vi "LS372_setup.vi"() -> (0 "error out":errorcluster caption="Fehler (Ausgang)")   [LabVIEW 2019]
uses:
  Instrument_Setup.vi
  Global/Global Variables/Data_Display_global.vi
  Equipment/Lake Shore 372/Lake Shore 372.lvlib
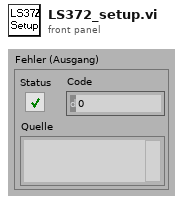
[diagram p1: front panel]
types:
  T1 = typedef "LS372-Cluster.ctl" = cluster{"Activate Tsweep":bool, "Setpoint - Manual":dbl, "Rate (K/min)":dbl, "Update Lakeshores":bool, "Still Heater":bool, "Still Power (mW)":dbl, "Manual Heater":bool, "Manual Heater  (mW) ":dbl, "Heater Range":dbl, "P (Gain)":dbl, "I (Reset)":dbl, "D (Rate)":dbl, "Heater Power (mW)":dbl, "MC Thermometer":u16, "MC Temperature":dbl, "LS372-T1":dbl, "LS372 -T2":dbl, "LS372-R1 ":dbl, "LS372-R2":dbl, "LS372-T3":dbl, "LS372-T4":dbl, "LS372-R3 ":dbl, "LS372-R4 \n\n\n\n":dbl, "LS372-T5":dbl, "LS372-T6":dbl, "LS372-R5":dbl, "LS372-R6 ":dbl, "Still Power ist":dbl, "Set Temperatur Sweep main":bool, "Setpoint ist":dbl, "Disable Heater":bool}
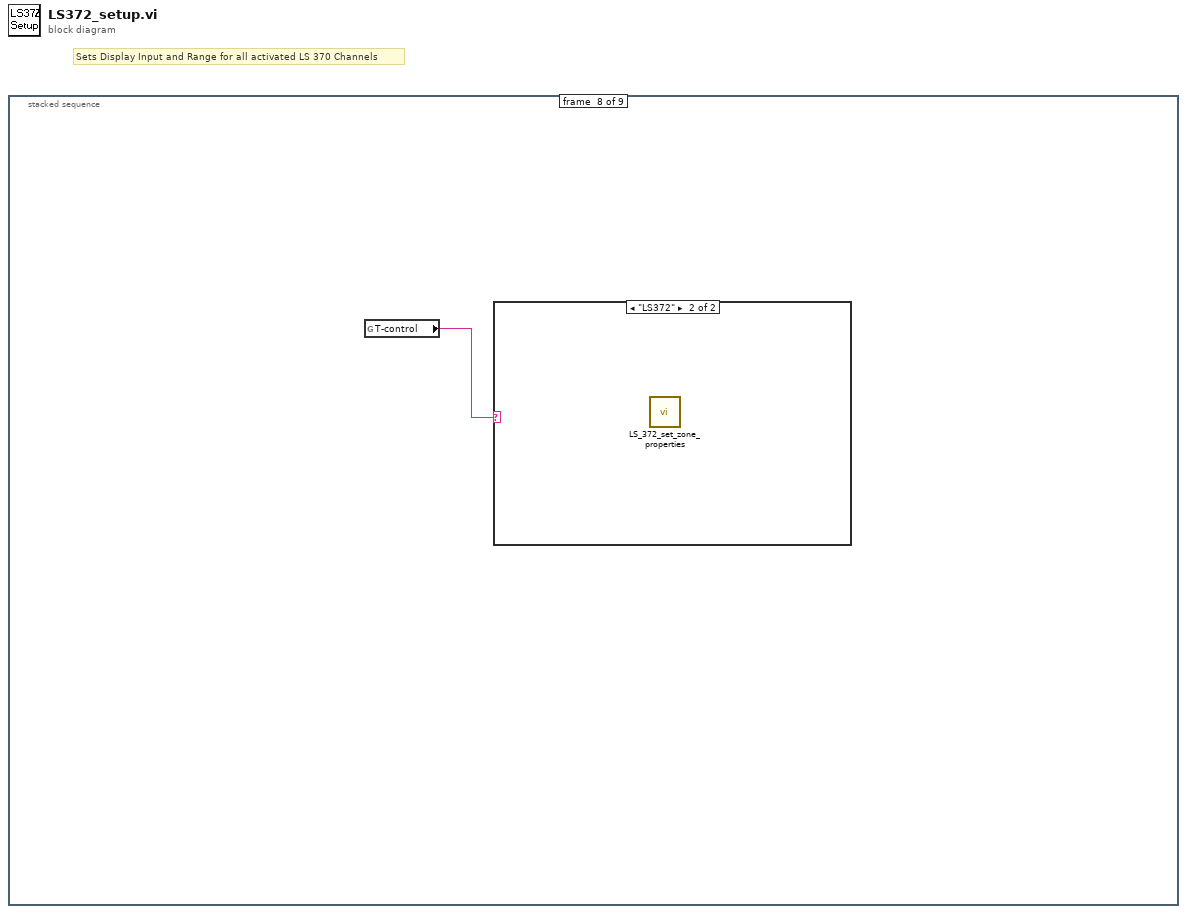
[diagram p0: block diagram]
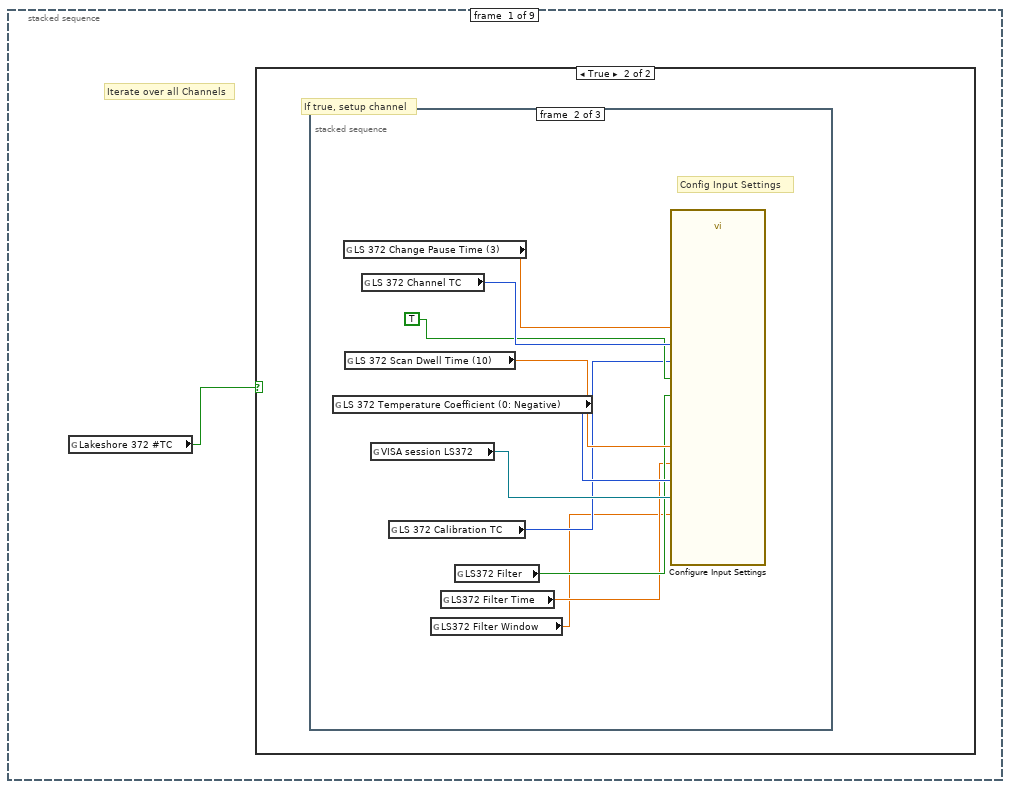
[diagram p2: hidden frame]
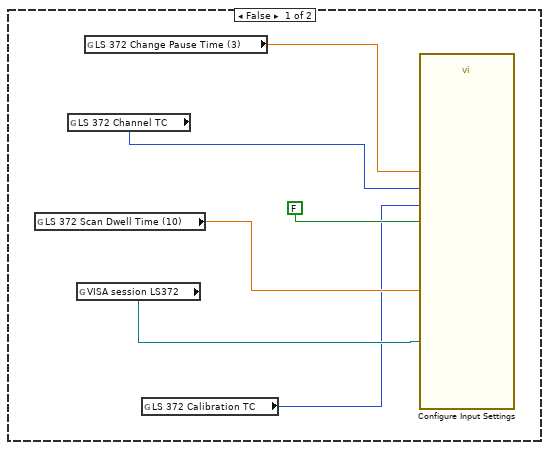
[diagram p3: hidden frame]
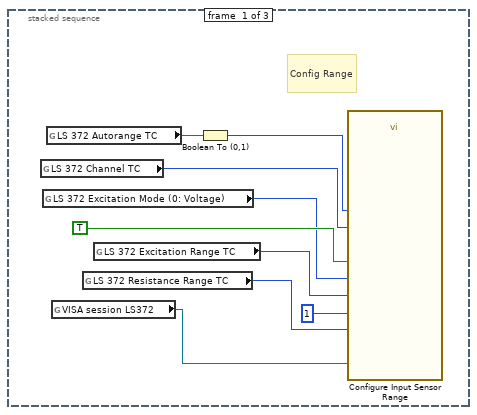
[diagram p4: hidden frame]
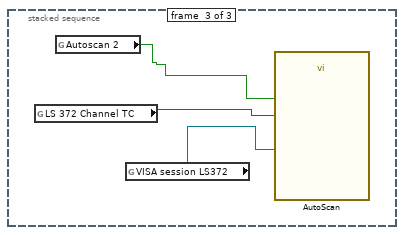
[diagram p5: hidden frame]
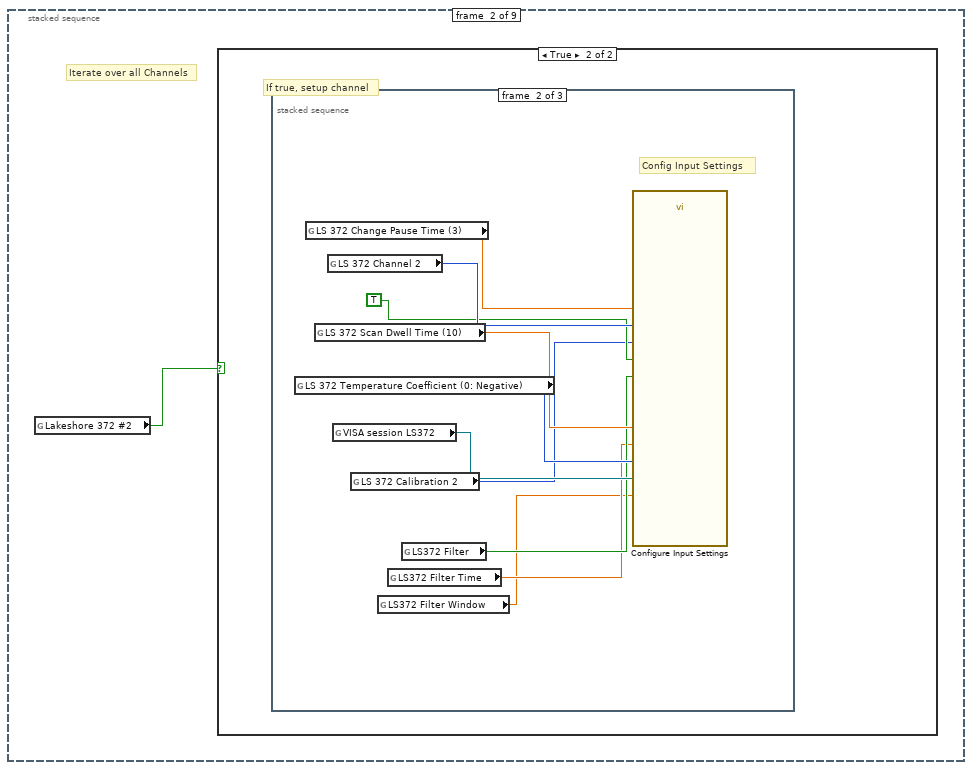
[diagram p6: hidden frame]
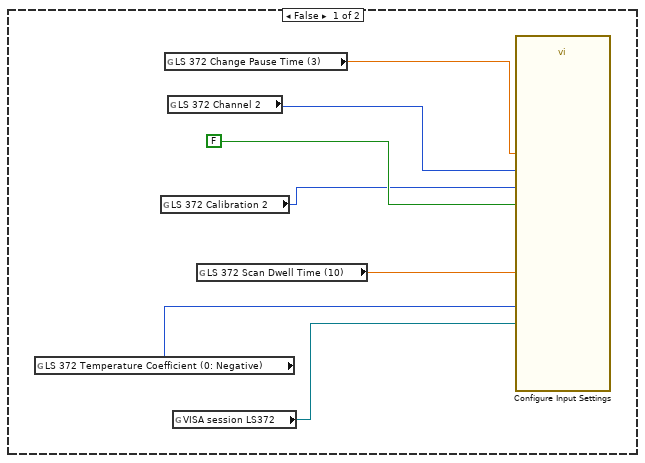
[diagram p7: hidden frame]
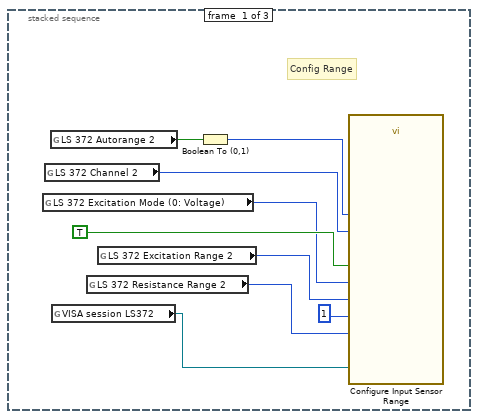
[diagram p8: hidden frame]
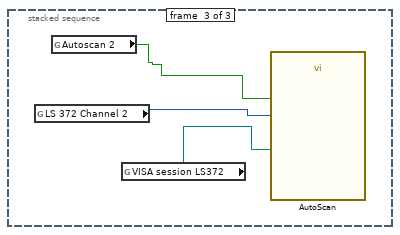
[diagram p9: hidden frame]
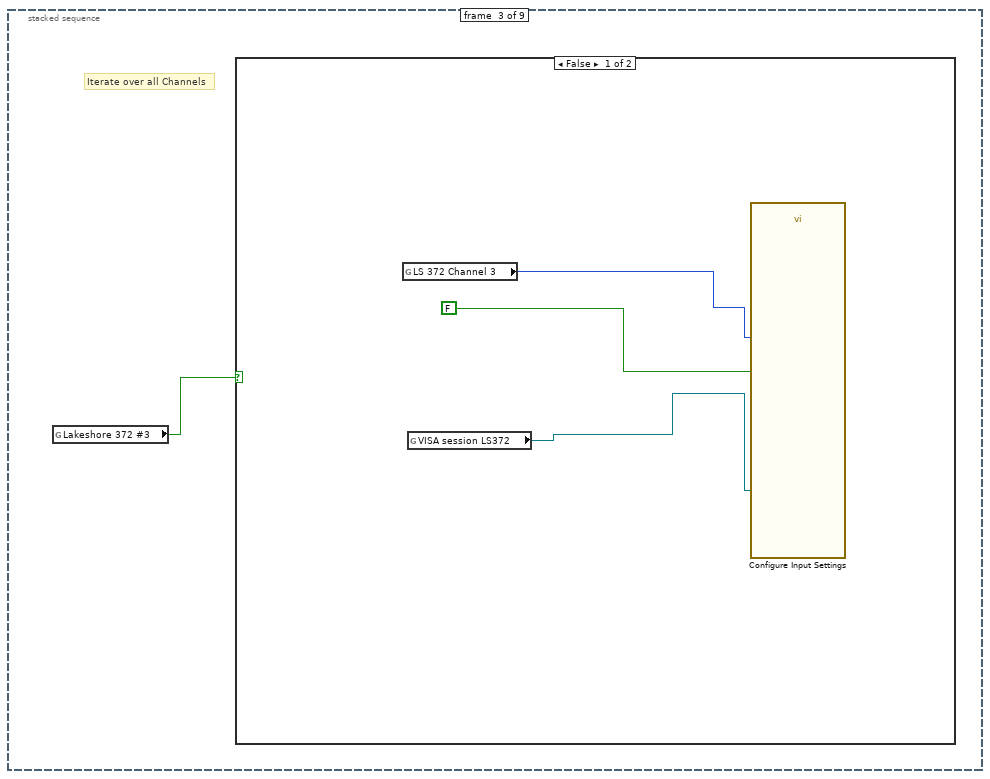
[diagram p10: hidden frame]
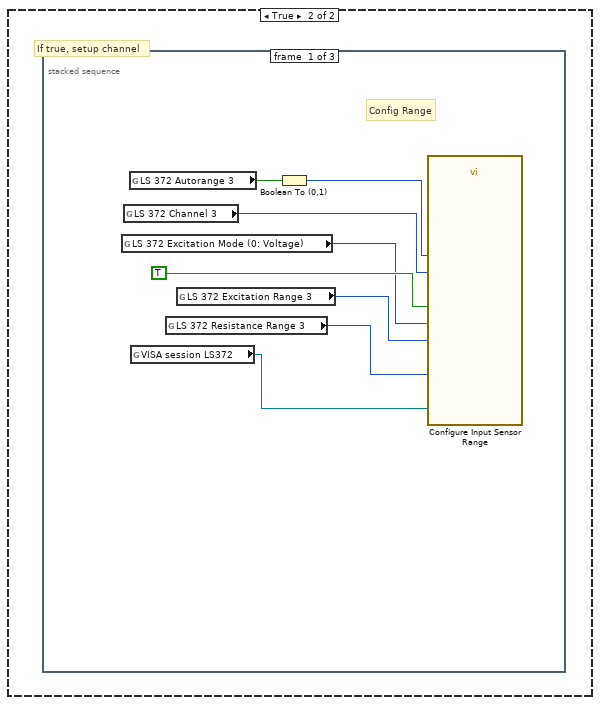
[diagram p11: hidden frame]
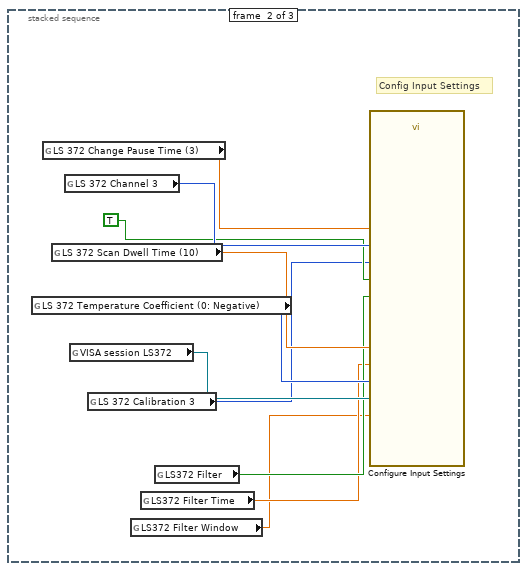
[diagram p12: hidden frame]
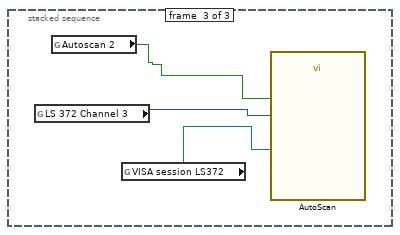
[diagram p13: hidden frame]
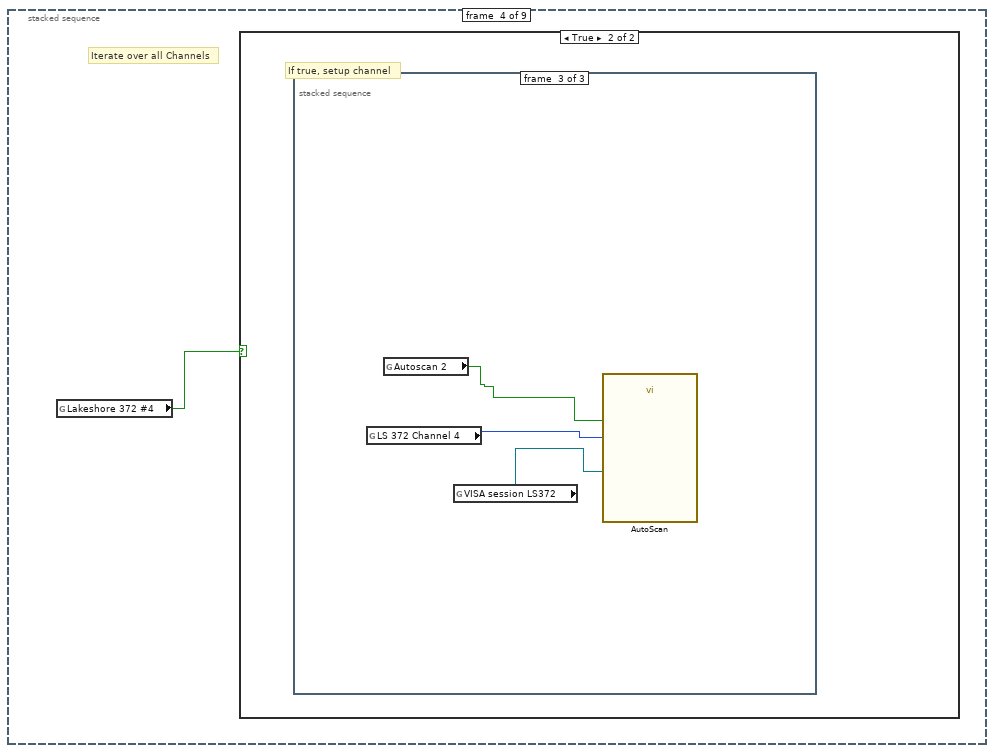
[diagram p14: hidden frame]
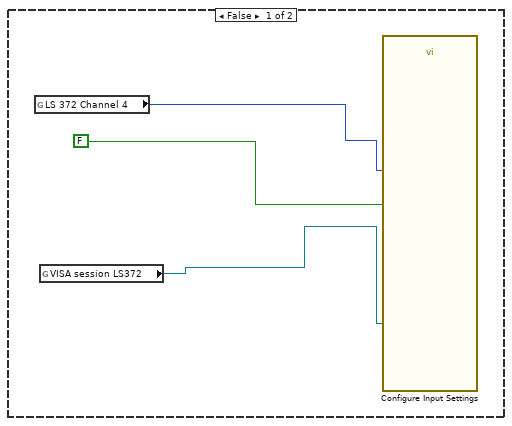
[diagram p15: hidden frame]
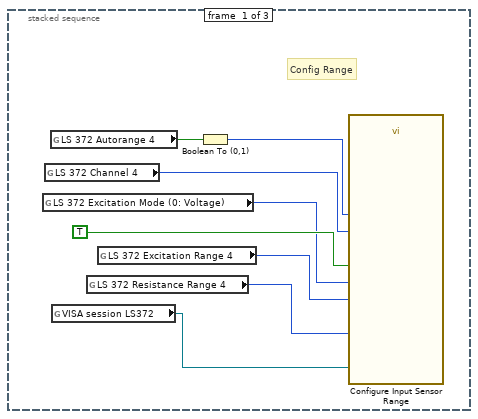
[diagram p16: hidden frame]
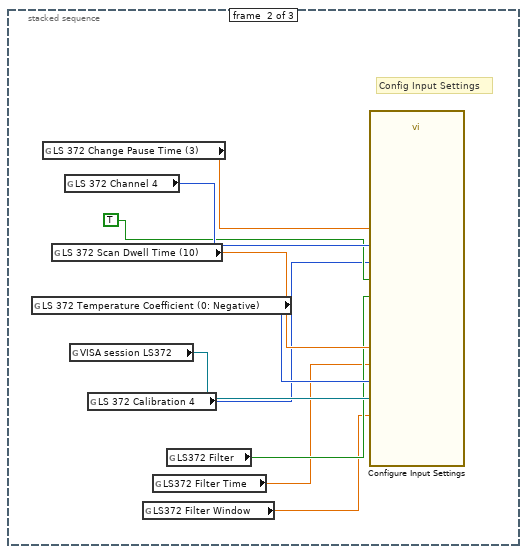
[diagram p17: hidden frame]
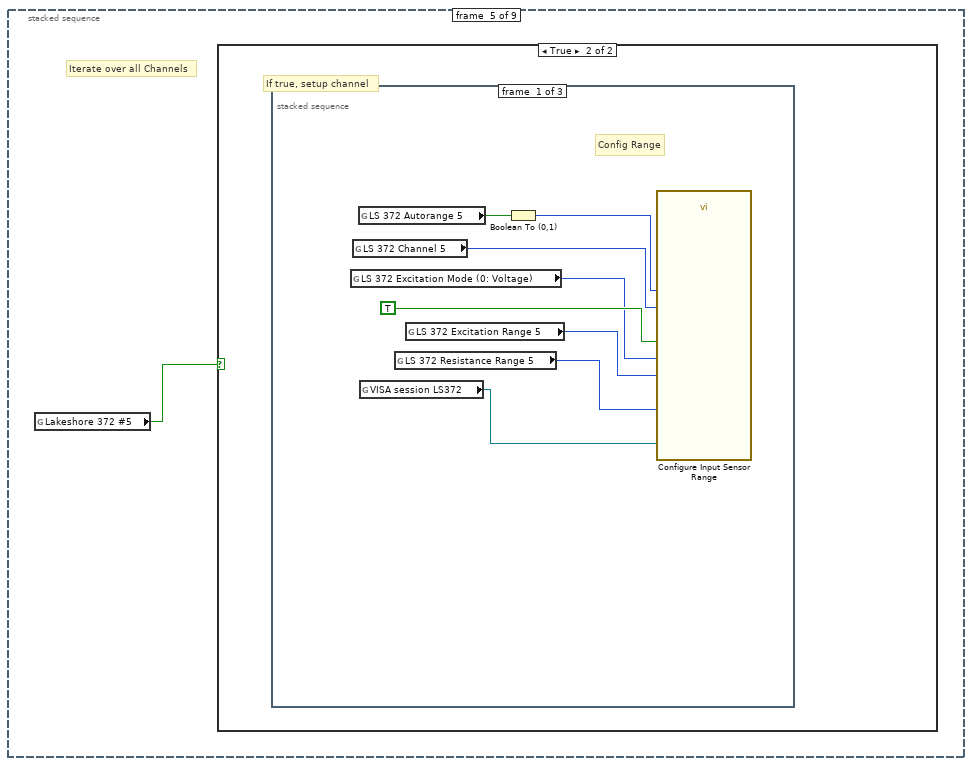
[diagram p18: hidden frame]
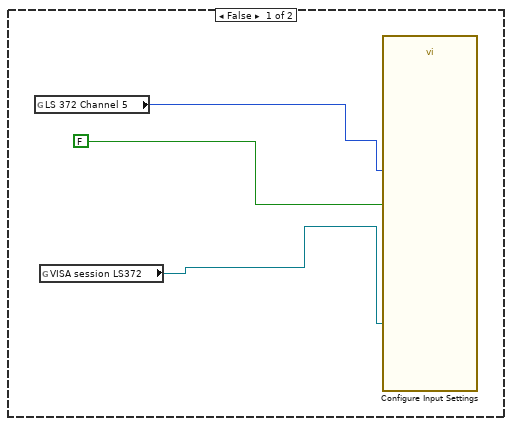
[diagram p19: hidden frame]
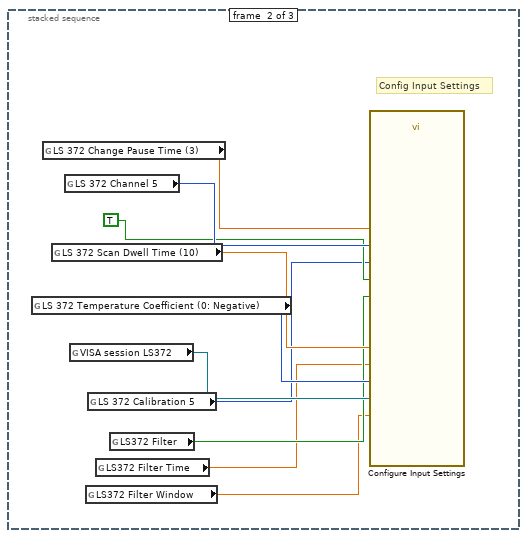
[diagram p20: hidden frame]
diagram:
  # "Sets Display Input and Range for all activated LS 370 Channels"
  n1 = stacked-sequence {
    frame #0 {
      # "Iterate over all Channels"
      n2 = global read "Instrument_Setup.vi" "Lakeshore 372 #TC"() -> (w1:bool)
      n3 = case shown="True" w1 {
        frame False {
          n4 = global read "Instrument_Setup.vi" "LS 372 Scan Dwell Time (10)"() -> (w3:dbl)
          n5 = global read "Instrument_Setup.vi" "LS 372 Channel TC"() -> (w7:u16)
          n6 = global read "Instrument_Setup.vi" "VISA session LS372"() -> (w5:refnum<visa-resource-name>)
          n7 = global read "Instrument_Setup.vi" "LS 372 Change Pause Time (3)"() -> (w4:dbl)
          n8 = global read "Instrument_Setup.vi" "LS 372 Calibration TC"() -> (w2:i32)
          n9 = call "Configure Input Settings.vi"("VISA resource name"=w5, "Channel (1)"=w7, "Scan Dwell Time (10)"=w3, "Change Pause Time (3)"=w4, "Curve Number (0)"=w2, "Enable Channel (T: Enable)"=FALSE) -> ()  [unwired: 12 in, 2 out]
        }
        frame True {
          # "If true, setup channel"
          n10 = stacked-sequence {
            frame #0 {
              # "Config Range"
              n11 = global read "Instrument_Setup.vi" "LS 372 Channel TC"() -> (w14:u16)
              n12 = global read "Instrument_Setup.vi" "LS 372 Excitation Mode (0: Voltage)"() -> (w12:u16)
              n13 = global read "Instrument_Setup.vi" "LS 372 Autorange TC"() -> (w16:bool)
              n14 = global read "Instrument_Setup.vi" "VISA session LS372"() -> (w9:refnum<visa-resource-name>)
              n15 = global read "Instrument_Setup.vi" "LS 372 Resistance Range TC"() -> (w10:u16)
              n16 = global read "Instrument_Setup.vi" "LS 372 Excitation Range TC"() -> (w11:u16)
              n17 = Boolean To (0,1)(Boolean=w16) -> (0, 1=w15:i16)
              n18 = call "Configure Input Sensor Range.vi"("VISA resource name"=w9, "Channel (1)"=w14, "Excitation Mode (0: Voltage)"=w12, "Excitation Range (5: 200 uV / 100 pA)"=w11, "Autorange (0: Autorange off)"=w15, "Resistance Range (17: 200 kOhm)"=w10, "Excitation  (T: On)"=TRUE, "Preferred Units (2: Ohms)"=1) -> ()  [unwired: 10 in, 2 out]
            }
            frame #1 {
              # "Config Input Settings"
              n19 = global read "Instrument_Setup.vi" "LS 372 Temperature Coefficient (0: Negative)"() -> (w22:u16)
              n20 = global read "Instrument_Setup.vi" "LS 372 Change Pause Time (3)"() -> (w26:dbl)
              n21 = global read "Instrument_Setup.vi" "LS 372 Scan Dwell Time (10)"() -> (w23:dbl)
              n22 = global read "Instrument_Setup.vi" "LS 372 Channel TC"() -> (w25:u16)
              n23 = global read "Instrument_Setup.vi" "VISA session LS372"() -> (w21:refnum<visa-resource-name>)
              n24 = global read "Instrument_Setup.vi" "LS 372 Calibration TC"() -> (w20:i32)
              n25 = global read "Instrument_Setup.vi" "LS372 Filter Window"() -> (w17:dbl)
              n26 = global read "Instrument_Setup.vi" "LS372 Filter Time"() -> (w18:dbl)
              n27 = global read "Instrument_Setup.vi" "LS372 Filter"() -> (w19:bool)
              n28 = call "Configure Input Settings.vi"("VISA resource name"=w21, "Channel (1)"=w25, "Scan Dwell Time (10)"=w23, "Change Pause Time (3)"=w26, "Curve Number (0)"=w20, "Enable Channel (T: Enable)"=TRUE, "Enable Filter (F: Off)"=w19, "Temperature Coefficient (1: Negative)"=w22, "Settle Time (10 sec)"=w18, "Window (40% FS)"=w17) -> ()  [unwired: 8 in, 2 out]
            }
            frame #2 {
              n29 = global read "Instrument_Setup.vi" "LS 372 Channel TC"() -> (w28:u16)
              n30 = global read "Instrument_Setup.vi" "Autoscan 2"() -> (w29:bool)
              n31 = global read "Instrument_Setup.vi" "VISA session LS372"() -> (w27:refnum<visa-resource-name>)
              n32 = call "AutoScan.vi"("Autoscan (F: Off)"=w29, "Channel (1:1)"=w28, "VISA resource name"=w27) -> ()  [unwired: 7 in, 2 out]
            }
          }
        }
      }
    }
    frame #1 {
      # "Iterate over all Channels"
      n33 = global read "Instrument_Setup.vi" "Lakeshore 372 #2"() -> (w30:bool)
      n34 = case shown="True" w30 {
        frame False {
          n35 = global read "Instrument_Setup.vi" "LS 372 Temperature Coefficient (0: Negative)"() -> (w33:u16)
          n36 = global read "Instrument_Setup.vi" "LS 372 Calibration 2"() -> (w32:i32)
          n37 = global read "Instrument_Setup.vi" "LS 372 Change Pause Time (3)"() -> (w34:dbl)
          n38 = global read "Instrument_Setup.vi" "LS 372 Channel 2"() -> (w37:u16)
          n39 = global read "Instrument_Setup.vi" "VISA session LS372"() -> (w35:refnum<visa-resource-name>)
          n40 = global read "Instrument_Setup.vi" "LS 372 Scan Dwell Time (10)"() -> (w31:dbl)
          n41 = call "Configure Input Settings.vi"("VISA resource name"=w35, "Channel (1)"=w37, "Scan Dwell Time (10)"=w31, "Change Pause Time (3)"=w34, "Curve Number (0)"=w32, "Enable Channel (T: Enable)"=FALSE, "Temperature Coefficient (1: Negative)"=w33) -> ()  [unwired: 11 in, 2 out]
        }
        frame True {
          # "If true, setup channel"
          n42 = stacked-sequence {
            frame #0 {
              # "Config Range"
              n43 = global read "Instrument_Setup.vi" "LS 372 Excitation Mode (0: Voltage)"() -> (w42:u16)
              n44 = global read "Instrument_Setup.vi" "LS 372 Channel 2"() -> (w44:u16)
              n45 = global read "Instrument_Setup.vi" "LS 372 Autorange 2"() -> (w46:bool)
              n46 = global read "Instrument_Setup.vi" "VISA session LS372"() -> (w39:refnum<visa-resource-name>)
              n47 = global read "Instrument_Setup.vi" "LS 372 Resistance Range 2"() -> (w40:u16)
              n48 = global read "Instrument_Setup.vi" "LS 372 Excitation Range 2"() -> (w41:u16)
              n49 = Boolean To (0,1)(Boolean=w46) -> (0, 1=w45:i16)
              n50 = call "Configure Input Sensor Range.vi"("VISA resource name"=w39, "Channel (1)"=w44, "Excitation Mode (0: Voltage)"=w42, "Excitation Range (5: 200 uV / 100 pA)"=w41, "Autorange (0: Autorange off)"=w45, "Resistance Range (17: 200 kOhm)"=w40, "Excitation  (T: On)"=TRUE, "Preferred Units (2: Ohms)"=1) -> ()  [unwired: 10 in, 2 out]
            }
            frame #1 {
              # "Config Input Settings"
              n51 = global read "Instrument_Setup.vi" "LS 372 Temperature Coefficient (0: Negative)"() -> (w52:u16)
              n52 = global read "Instrument_Setup.vi" "LS 372 Change Pause Time (3)"() -> (w56:dbl)
              n53 = global read "Instrument_Setup.vi" "LS 372 Scan Dwell Time (10)"() -> (w53:dbl)
              n54 = global read "Instrument_Setup.vi" "LS 372 Channel 2"() -> (w55:u16)
              n55 = global read "Instrument_Setup.vi" "VISA session LS372"() -> (w51:refnum<visa-resource-name>)
              n56 = global read "Instrument_Setup.vi" "LS 372 Calibration 2"() -> (w50:i32)
              n57 = global read "Instrument_Setup.vi" "LS372 Filter Window"() -> (w47:dbl)
              n58 = global read "Instrument_Setup.vi" "LS372 Filter Time"() -> (w48:dbl)
              n59 = global read "Instrument_Setup.vi" "LS372 Filter"() -> (w49:bool)
              n60 = call "Configure Input Settings.vi"("VISA resource name"=w51, "Channel (1)"=w55, "Scan Dwell Time (10)"=w53, "Change Pause Time (3)"=w56, "Curve Number (0)"=w50, "Enable Channel (T: Enable)"=TRUE, "Enable Filter (F: Off)"=w49, "Temperature Coefficient (1: Negative)"=w52, "Settle Time (10 sec)"=w48, "Window (40% FS)"=w47) -> ()  [unwired: 8 in, 2 out]
            }
            frame #2 {
              n61 = global read "Instrument_Setup.vi" "LS 372 Channel 2"() -> (w58:u16)
              n62 = global read "Instrument_Setup.vi" "Autoscan 2"() -> (w59:bool)
              n63 = global read "Instrument_Setup.vi" "VISA session LS372"() -> (w57:refnum<visa-resource-name>)
              n64 = call "AutoScan.vi"("Autoscan (F: Off)"=w59, "Channel (1:1)"=w58, "VISA resource name"=w57) -> ()  [unwired: 7 in, 2 out]
            }
          }
        }
      }
    }
    frame #2 {
      # "Iterate over all Channels"
      n65 = global read "Instrument_Setup.vi" "Lakeshore 372 #3"() -> (w60:bool)
      n66 = case shown="False" w60 {
        frame False {
          n67 = global read "Instrument_Setup.vi" "LS 372 Channel 3"() -> (w63:u16)
          n68 = global read "Instrument_Setup.vi" "VISA session LS372"() -> (w61:refnum<visa-resource-name>)
          n69 = call "Configure Input Settings.vi"("VISA resource name"=w61, "Channel (1)"=w63, "Enable Channel (T: Enable)"=FALSE) -> ()  [unwired: 15 in, 2 out]
        }
        frame True {
          # "If true, setup channel"
          n70 = stacked-sequence {
            frame #0 {
              # "Config Range"
              n71 = global read "Instrument_Setup.vi" "LS 372 Excitation Mode (0: Voltage)"() -> (w67:u16)
              n72 = global read "Instrument_Setup.vi" "LS 372 Channel 3"() -> (w69:u16)
              n73 = global read "Instrument_Setup.vi" "LS 372 Autorange 3"() -> (w71:bool)
              n74 = global read "Instrument_Setup.vi" "VISA session LS372"() -> (w64:refnum<visa-resource-name>)
              n75 = global read "Instrument_Setup.vi" "LS 372 Resistance Range 3"() -> (w65:u16)
              n76 = global read "Instrument_Setup.vi" "LS 372 Excitation Range 3"() -> (w66:u16)
              n77 = Boolean To (0,1)(Boolean=w71) -> (0, 1=w70:i16)
              n78 = call "Configure Input Sensor Range.vi"("VISA resource name"=w64, "Channel (1)"=w69, "Excitation Mode (0: Voltage)"=w67, "Excitation Range (5: 200 uV / 100 pA)"=w66, "Autorange (0: Autorange off)"=w70, "Resistance Range (17: 200 kOhm)"=w65, "Excitation  (T: On)"=TRUE) -> ()  [unwired: 11 in, 2 out]
            }
            frame #1 {
              # "Config Input Settings"
              n79 = global read "Instrument_Setup.vi" "LS 372 Temperature Coefficient (0: Negative)"() -> (w77:u16)
              n80 = global read "Instrument_Setup.vi" "LS 372 Change Pause Time (3)"() -> (w81:dbl)
              n81 = global read "Instrument_Setup.vi" "LS 372 Scan Dwell Time (10)"() -> (w78:dbl)
              n82 = global read "Instrument_Setup.vi" "LS 372 Channel 3"() -> (w80:u16)
              n83 = global read "Instrument_Setup.vi" "VISA session LS372"() -> (w76:refnum<visa-resource-name>)
              n84 = global read "Instrument_Setup.vi" "LS 372 Calibration 3"() -> (w75:i32)
              n85 = global read "Instrument_Setup.vi" "LS372 Filter Window"() -> (w72:dbl)
              n86 = global read "Instrument_Setup.vi" "LS372 Filter Time"() -> (w73:dbl)
              n87 = global read "Instrument_Setup.vi" "LS372 Filter"() -> (w74:bool)
              n88 = call "Configure Input Settings.vi"("VISA resource name"=w76, "Channel (1)"=w80, "Scan Dwell Time (10)"=w78, "Change Pause Time (3)"=w81, "Curve Number (0)"=w75, "Enable Channel (T: Enable)"=TRUE, "Enable Filter (F: Off)"=w74, "Temperature Coefficient (1: Negative)"=w77, "Settle Time (10 sec)"=w73, "Window (40% FS)"=w72) -> ()  [unwired: 8 in, 2 out]
            }
            frame #2 {
              n89 = global read "Instrument_Setup.vi" "LS 372 Channel 3"() -> (w83:u16)
              n90 = global read "Instrument_Setup.vi" "Autoscan 2"() -> (w84:bool)
              n91 = global read "Instrument_Setup.vi" "VISA session LS372"() -> (w82:refnum<visa-resource-name>)
              n92 = call "AutoScan.vi"("Autoscan (F: Off)"=w84, "Channel (1:1)"=w83, "VISA resource name"=w82) -> ()  [unwired: 7 in, 2 out]
            }
          }
        }
      }
    }
    frame #3 {
      # "Iterate over all Channels"
      n93 = global read "Instrument_Setup.vi" "Lakeshore 372 #4"() -> (w85:bool)
      n94 = case shown="True" w85 {
        frame False {
          n95 = global read "Instrument_Setup.vi" "LS 372 Channel 4"() -> (w88:u16)
          n96 = global read "Instrument_Setup.vi" "VISA session LS372"() -> (w86:refnum<visa-resource-name>)
          n97 = call "Configure Input Settings.vi"("VISA resource name"=w86, "Channel (1)"=w88, "Enable Channel (T: Enable)"=FALSE) -> ()  [unwired: 15 in, 2 out]
        }
        frame True {
          # "If true, setup channel"
          n98 = stacked-sequence {
            frame #0 {
              # "Config Range"
              n99 = global read "Instrument_Setup.vi" "LS 372 Excitation Mode (0: Voltage)"() -> (w92:u16)
              n100 = global read "Instrument_Setup.vi" "LS 372 Channel 4"() -> (w94:u16)
              n101 = global read "Instrument_Setup.vi" "LS 372 Autorange 4"() -> (w96:bool)
              n102 = global read "Instrument_Setup.vi" "VISA session LS372"() -> (w89:refnum<visa-resource-name>)
              n103 = global read "Instrument_Setup.vi" "LS 372 Resistance Range 4"() -> (w90:u16)
              n104 = global read "Instrument_Setup.vi" "LS 372 Excitation Range 4"() -> (w91:u16)
              n105 = Boolean To (0,1)(Boolean=w96) -> (0, 1=w95:i16)
              n106 = call "Configure Input Sensor Range.vi"("VISA resource name"=w89, "Channel (1)"=w94, "Excitation Mode (0: Voltage)"=w92, "Excitation Range (5: 200 uV / 100 pA)"=w91, "Autorange (0: Autorange off)"=w95, "Resistance Range (17: 200 kOhm)"=w90, "Excitation  (T: On)"=TRUE) -> ()  [unwired: 11 in, 2 out]
            }
            frame #1 {
              # "Config Input Settings"
              n107 = global read "Instrument_Setup.vi" "LS 372 Temperature Coefficient (0: Negative)"() -> (w102:u16)
              n108 = global read "Instrument_Setup.vi" "LS 372 Change Pause Time (3)"() -> (w106:dbl)
              n109 = global read "Instrument_Setup.vi" "LS 372 Scan Dwell Time (10)"() -> (w103:dbl)
              n110 = global read "Instrument_Setup.vi" "LS 372 Channel 4"() -> (w105:u16)
              n111 = global read "Instrument_Setup.vi" "VISA session LS372"() -> (w101:refnum<visa-resource-name>)
              n112 = global read "Instrument_Setup.vi" "LS 372 Calibration 4"() -> (w100:i32)
              n113 = global read "Instrument_Setup.vi" "LS372 Filter Window"() -> (w97:dbl)
              n114 = global read "Instrument_Setup.vi" "LS372 Filter Time"() -> (w98:dbl)
              n115 = global read "Instrument_Setup.vi" "LS372 Filter"() -> (w99:bool)
              n116 = call "Configure Input Settings.vi"("VISA resource name"=w101, "Channel (1)"=w105, "Scan Dwell Time (10)"=w103, "Change Pause Time (3)"=w106, "Curve Number (0)"=w100, "Enable Channel (T: Enable)"=TRUE, "Enable Filter (F: Off)"=w99, "Temperature Coefficient (1: Negative)"=w102, "Settle Time (10 sec)"=w98, "Window (40% FS)"=w97) -> ()  [unwired: 8 in, 2 out]
            }
            frame #2 {
              n117 = global read "Instrument_Setup.vi" "LS 372 Channel 4"() -> (w108:u16)
              n118 = global read "Instrument_Setup.vi" "Autoscan 2"() -> (w109:bool)
              n119 = global read "Instrument_Setup.vi" "VISA session LS372"() -> (w107:refnum<visa-resource-name>)
              n120 = call "AutoScan.vi"("Autoscan (F: Off)"=w109, "Channel (1:1)"=w108, "VISA resource name"=w107) -> ()  [unwired: 7 in, 2 out]
            }
          }
        }
      }
    }
    frame #4 {
      # "Iterate over all Channels"
      n121 = global read "Instrument_Setup.vi" "Lakeshore 372 #5"() -> (w110:bool)
      n122 = case shown="True" w110 {
        frame False {
          n123 = global read "Instrument_Setup.vi" "LS 372 Channel 5"() -> (w113:u16)
          n124 = global read "Instrument_Setup.vi" "VISA session LS372"() -> (w111:refnum<visa-resource-name>)
          n125 = call "Configure Input Settings.vi"("VISA resource name"=w111, "Channel (1)"=w113, "Enable Channel (T: Enable)"=FALSE) -> ()  [unwired: 15 in, 2 out]
        }
        frame True {
          # "If true, setup channel"
          n126 = stacked-sequence {
            frame #0 {
              # "Config Range"
              n127 = global read "Instrument_Setup.vi" "LS 372 Excitation Mode (0: Voltage)"() -> (w117:u16)
              n128 = global read "Instrument_Setup.vi" "LS 372 Channel 5"() -> (w119:u16)
              n129 = global read "Instrument_Setup.vi" "LS 372 Autorange 5"() -> (w121:bool)
              n130 = global read "Instrument_Setup.vi" "VISA session LS372"() -> (w114:refnum<visa-resource-name>)
              n131 = global read "Instrument_Setup.vi" "LS 372 Resistance Range 5"() -> (w115:u16)
              n132 = global read "Instrument_Setup.vi" "LS 372 Excitation Range 5"() -> (w116:u16)
              n133 = Boolean To (0,1)(Boolean=w121) -> (0, 1=w120:i16)
              n134 = call "Configure Input Sensor Range.vi"("VISA resource name"=w114, "Channel (1)"=w119, "Excitation Mode (0: Voltage)"=w117, "Excitation Range (5: 200 uV / 100 pA)"=w116, "Autorange (0: Autorange off)"=w120, "Resistance Range (17: 200 kOhm)"=w115, "Excitation  (T: On)"=TRUE) -> ()  [unwired: 11 in, 2 out]
            }
            frame #1 {
              # "Config Input Settings"
              n135 = global read "Instrument_Setup.vi" "LS 372 Temperature Coefficient (0: Negative)"() -> (w127:u16)
              n136 = global read "Instrument_Setup.vi" "LS 372 Change Pause Time (3)"() -> (w131:dbl)
              n137 = global read "Instrument_Setup.vi" "LS 372 Scan Dwell Time (10)"() -> (w128:dbl)
              n138 = global read "Instrument_Setup.vi" "LS 372 Channel 5"() -> (w130:u16)
              n139 = global read "Instrument_Setup.vi" "VISA session LS372"() -> (w126:refnum<visa-resource-name>)
              n140 = global read "Instrument_Setup.vi" "LS372 Filter Window"() -> (w122:dbl)
              n141 = global read "Instrument_Setup.vi" "LS 372 Calibration 5"() -> (w125:i32)
              n142 = global read "Instrument_Setup.vi" "LS372 Filter Time"() -> (w123:dbl)
              n143 = global read "Instrument_Setup.vi" "LS372 Filter"() -> (w124:bool)
              n144 = call "Configure Input Settings.vi"("VISA resource name"=w126, "Channel (1)"=w130, "Scan Dwell Time (10)"=w128, "Change Pause Time (3)"=w131, "Curve Number (0)"=w125, "Enable Channel (T: Enable)"=TRUE, "Enable Filter (F: Off)"=w124, "Temperature Coefficient (1: Negative)"=w127, "Settle Time (10 sec)"=w123, "Window (40% FS)"=w122) -> ()  [unwired: 8 in, 2 out]
            }
            frame #2 {
              n145 = global read "Instrument_Setup.vi" "LS 372 Channel 5"() -> (w133:u16)
              n146 = global read "Instrument_Setup.vi" "Autoscan 2"() -> (w134:bool)
              n147 = global read "Instrument_Setup.vi" "VISA session LS372"() -> (w132:refnum<visa-resource-name>)
              n148 = call "AutoScan.vi"("Autoscan (F: Off)"=w134, "Channel (1:1)"=w133, "VISA resource name"=w132) -> ()  [unwired: 7 in, 2 out]
            }
          }
        }
      }
    }
    frame #5 {
      # "Iterate over all Channels"
      n149 = global read "Instrument_Setup.vi" "Lakeshore 372 #6"() -> (w135:bool)
      n150 = case shown="True" w135 {
        frame False {
          n151 = global read "Instrument_Setup.vi" "LS 372 Channel 6"() -> (w138:u16)
          n152 = global read "Instrument_Setup.vi" "VISA session LS372"() -> (w136:refnum<visa-resource-name>)
          n153 = call "Configure Input Settings.vi"("VISA resource name"=w136, "Channel (1)"=w138, "Enable Channel (T: Enable)"=FALSE) -> ()  [unwired: 15 in, 2 out]
        }
        frame True {
          # "If true, setup channel"
          n154 = stacked-sequence {
            frame #0 {
              # "Config Range"
              n155 = global read "Instrument_Setup.vi" "LS 372 Excitation Mode (0: Voltage)"() -> (w142:u16)
              n156 = global read "Instrument_Setup.vi" "LS 372 Channel 6"() -> (w144:u16)
              n157 = global read "Instrument_Setup.vi" "LS 372  Autorange 6"() -> (w146:bool)
              n158 = global read "Instrument_Setup.vi" "VISA session LS372"() -> (w139:refnum<visa-resource-name>)
              n159 = global read "Instrument_Setup.vi" "LS 372 Resistance Range 6"() -> (w140:u16)
              n160 = global read "Instrument_Setup.vi" "LS 372 Excitation Range 6"() -> (w141:u16)
              n161 = Boolean To (0,1)(Boolean=w146) -> (0, 1=w145:i16)
              n162 = call "Configure Input Sensor Range.vi"("VISA resource name"=w139, "Channel (1)"=w144, "Excitation Mode (0: Voltage)"=w142, "Excitation Range (5: 200 uV / 100 pA)"=w141, "Autorange (0: Autorange off)"=w145, "Resistance Range (17: 200 kOhm)"=w140, "Excitation  (T: On)"=TRUE) -> ()  [unwired: 11 in, 2 out]
            }
            frame #1 {
              # "Config Input Settings"
              n163 = global read "Instrument_Setup.vi" "LS 372 Temperature Coefficient (0: Negative)"() -> (w152:u16)
              n164 = global read "Instrument_Setup.vi" "LS 372 Change Pause Time (3)"() -> (w156:dbl)
              n165 = global read "Instrument_Setup.vi" "LS 372 Scan Dwell Time (10)"() -> (w153:dbl)
              n166 = global read "Instrument_Setup.vi" "LS 372 Channel 6"() -> (w155:u16)
              n167 = global read "Instrument_Setup.vi" "VISA session LS372"() -> (w151:refnum<visa-resource-name>)
              n168 = global read "Instrument_Setup.vi" "LS 372 Calibration 6"() -> (w150:i32)
              n169 = global read "Instrument_Setup.vi" "LS372 Filter Window"() -> (w147:dbl)
              n170 = global read "Instrument_Setup.vi" "LS372 Filter Time"() -> (w148:dbl)
              n171 = global read "Instrument_Setup.vi" "LS372 Filter"() -> (w149:bool)
              n172 = call "Configure Input Settings.vi"("VISA resource name"=w151, "Channel (1)"=w155, "Scan Dwell Time (10)"=w153, "Change Pause Time (3)"=w156, "Curve Number (0)"=w150, "Enable Channel (T: Enable)"=TRUE, "Enable Filter (F: Off)"=w149, "Temperature Coefficient (1: Negative)"=w152, "Settle Time (10 sec)"=w148, "Window (40% FS)"=w147) -> ()  [unwired: 8 in, 2 out]
            }
            frame #2 {
              n173 = global read "Instrument_Setup.vi" "LS 372 Channel 6"() -> (w158:u16)
              n174 = global read "Instrument_Setup.vi" "Autoscan 2"() -> (w159:bool)
              n175 = global read "Instrument_Setup.vi" "VISA session LS372"() -> (w157:refnum<visa-resource-name>)
              n176 = call "AutoScan.vi"("Autoscan (F: Off)"=w159, "Channel (1:1)"=w158, "VISA resource name"=w157) -> ()  [unwired: 7 in, 2 out]
            }
          }
        }
      }
    }
    frame #6 {
      n177 = global read "Instrument_Setup.vi" "VISA session LS372"() -> (w161:refnum<visa-resource-name>)
      n178 = for {
        N: 11 -> [_]
        tunnel: w161 -> [w166]
        i -> [w163]
        n179 = Add(x=7, y=w163) -> (x+y=w162:i32)
        n180 = call "Configure Input Settings.vi"("VISA resource name"=w166, "Channel (1)"=w162, "Enable Channel (T: Enable)"=FALSE) -> ()  [unwired: 15 in, 2 out]
      }
    }
    frame #7 {
      n181 = global read "Instrument_Setup.vi" "T-control"() -> (w167:string)
      n182 = case shown="\"LS372\"" w167 {
        frame "None", Default {
        }
        frame "LS372" {
          n183 = call "LS_372_set_zone_properties.vi"() -> ()  [unwired: 12 in]
        }
      }
    }
    frame #8 {
      n184 = global read "Instrument_Setup.vi" "T-control"() -> (w168:string)
      n185 = case shown="\"LS372\"" w168 {
        frame "None", Default {
        }
        frame "LS372" {
          w172 = u16 0 items=["Auto off", "Continuous"] ("Warmup Control (0: Auto off)")
          w174 = u16 0 items=["Unipolar", "Bipolar"] ("Polarity (0: Unipolar)")
          w175 = u16 0 items=["Unfiltered", "Filtered"] ("Filtered Readings (0: Unfiltered)")
          w176 = u16 0 items=["sample heater", "output 1 (warm-up heater) ", "output 2 (analog/still)"] ("Output (0: sample heater)")
          w177 = u16 3 items=["Off", "Monitor Out", "Open Loop (Manual)", "Zone", "Still", "Closed Loop (PID)", "Warm-up"] ("Output Mode (0: Off)")
          # "Set Zone Tuning"
          n186 = global read "Data_Display_global.vi" "LS372-Cluster"() -> (w181:T1)
          n187 = Unbundle By Name(w181) -> ("MC Thermometer"=w180:u16)
          n188 = case shown="0, Default" w180 {
            tunnel: [w183 w184] -> w179
            frame 0, Default {
              n189 = global read "Instrument_Setup.vi" "LS 372 Channel TC"() -> (w183:u16)
            }
            frame 1 {
              n190 = global read "Instrument_Setup.vi" "LS 372 Channel 2"() -> (w184:u16)
            }
          }
          n191 = global read "Instrument_Setup.vi" "VISA session LS372"() -> (w170:refnum<visa-resource-name>)
          n192 = Wait (ms)(milliseconds to wait=1) -> ()  [unwired: 1 out]
          n193 = call "Configure Control Mode.vi"("VISA resource name"=w170, "Enable Power-up (F: Disable)"=FALSE, "Setpoint Change Delay (25sec)"=25, "Output (0: sample heater)"=w176, "Channel (1:1)"=w179, "Output Mode (0: Off)"=w177, "Polarity (0: Unipolar)"=w174, "Filtered Readings (0: Unfiltered)"=w175, "Warmup Control (0: Auto off)"=w172, "Warmup % (50%)"=50.0) -> ("error out"=→"error out":errorcluster)  [unwired: 4 in, 1 out]
        }
      }
    }
  }
